vi "Get AI Channel Name.vi"(8 "Error In":errorcluster, 10 "AI Channel Nums":u8[](array[numeric])) -> (0 "Error Out":errorcluster, 2 "AI Channels":string[](array[string]))   [LabVIEW 2011, in "LVH-LINX.lvlib" / "myRIO.lvlib"]
doc: "Get AI channel names (strings) from channel numbers."
uses:
  myRIO.lvlib
  Type Defs/AI Channel.ctl
panel:
  in  "AI Channel":T1
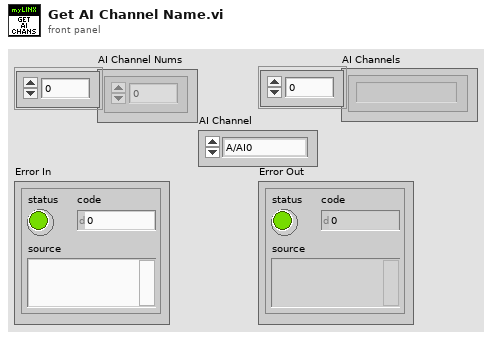
[diagram p1: front panel]
types:
  T1 = typedef "LVH-LINX.lvlib/myRIO.lvlib/AI Channel.ctl" = enum16{"A/AI0", "A/AI1", "A/AI2", "A/AI3", "B/AI0", "B/AI1", "B/AI2", "B/AI3", "C/AI0", "C/AI1"}
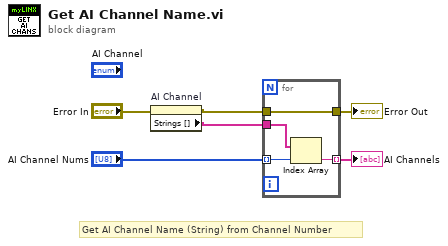
[diagram p0: block diagram]
diagram:
  # "Get AI Channel Name (String) from Channel Number"
  n1 = property on="AI Channel" class="Enum (strict)"(error in="Error In") -> (error out=w2:errorcluster, "Strings []"=w1:string[])  [unwired: 1 in, 1 out]
  n2 = for {
    tunnel: [w10] -> w6
    tunnel: w2 -> [w10]
    tunnel: w1 -> [w9]
    tunnel: "AI Channel Nums" -> [w8] mode=indexing
    tunnel: [w7] -> w4 mode=indexing
    n3 = Index Array(array=w9, index=w8) -> (element=w7:string)
  }
  "Error Out" <- w6
  "AI Channels" <- w4
